vi "OcsWriteFormCsv.vi"() -> ()   [LabVIEW 2018]
panel:
  out "Numeric":i32
  in  "Error in":errorcluster
  out "Error out":errorcluster
  out "W3-TESTER":string
  out "W8-TEXT4":string
  out "W9-OPNAME":string
  out "W0-SN 2":string
  out "SQL Execute":string="SELECT * FROM [FCTDATA].[dbo].[ABF]\nWHERE Barcode = 'P1813J0001'\nORDER BY ID"
  out "W0-SN":string
  out "element":i32
  out "array":string[][](array[string])
  in  ".csv":path
  out "Out":string
  in  "opname":string(combo)="FCT1"
  out "Start Time":dbl
  out "Sec":dbl
  # "Password:Abcd1234* 20220627"
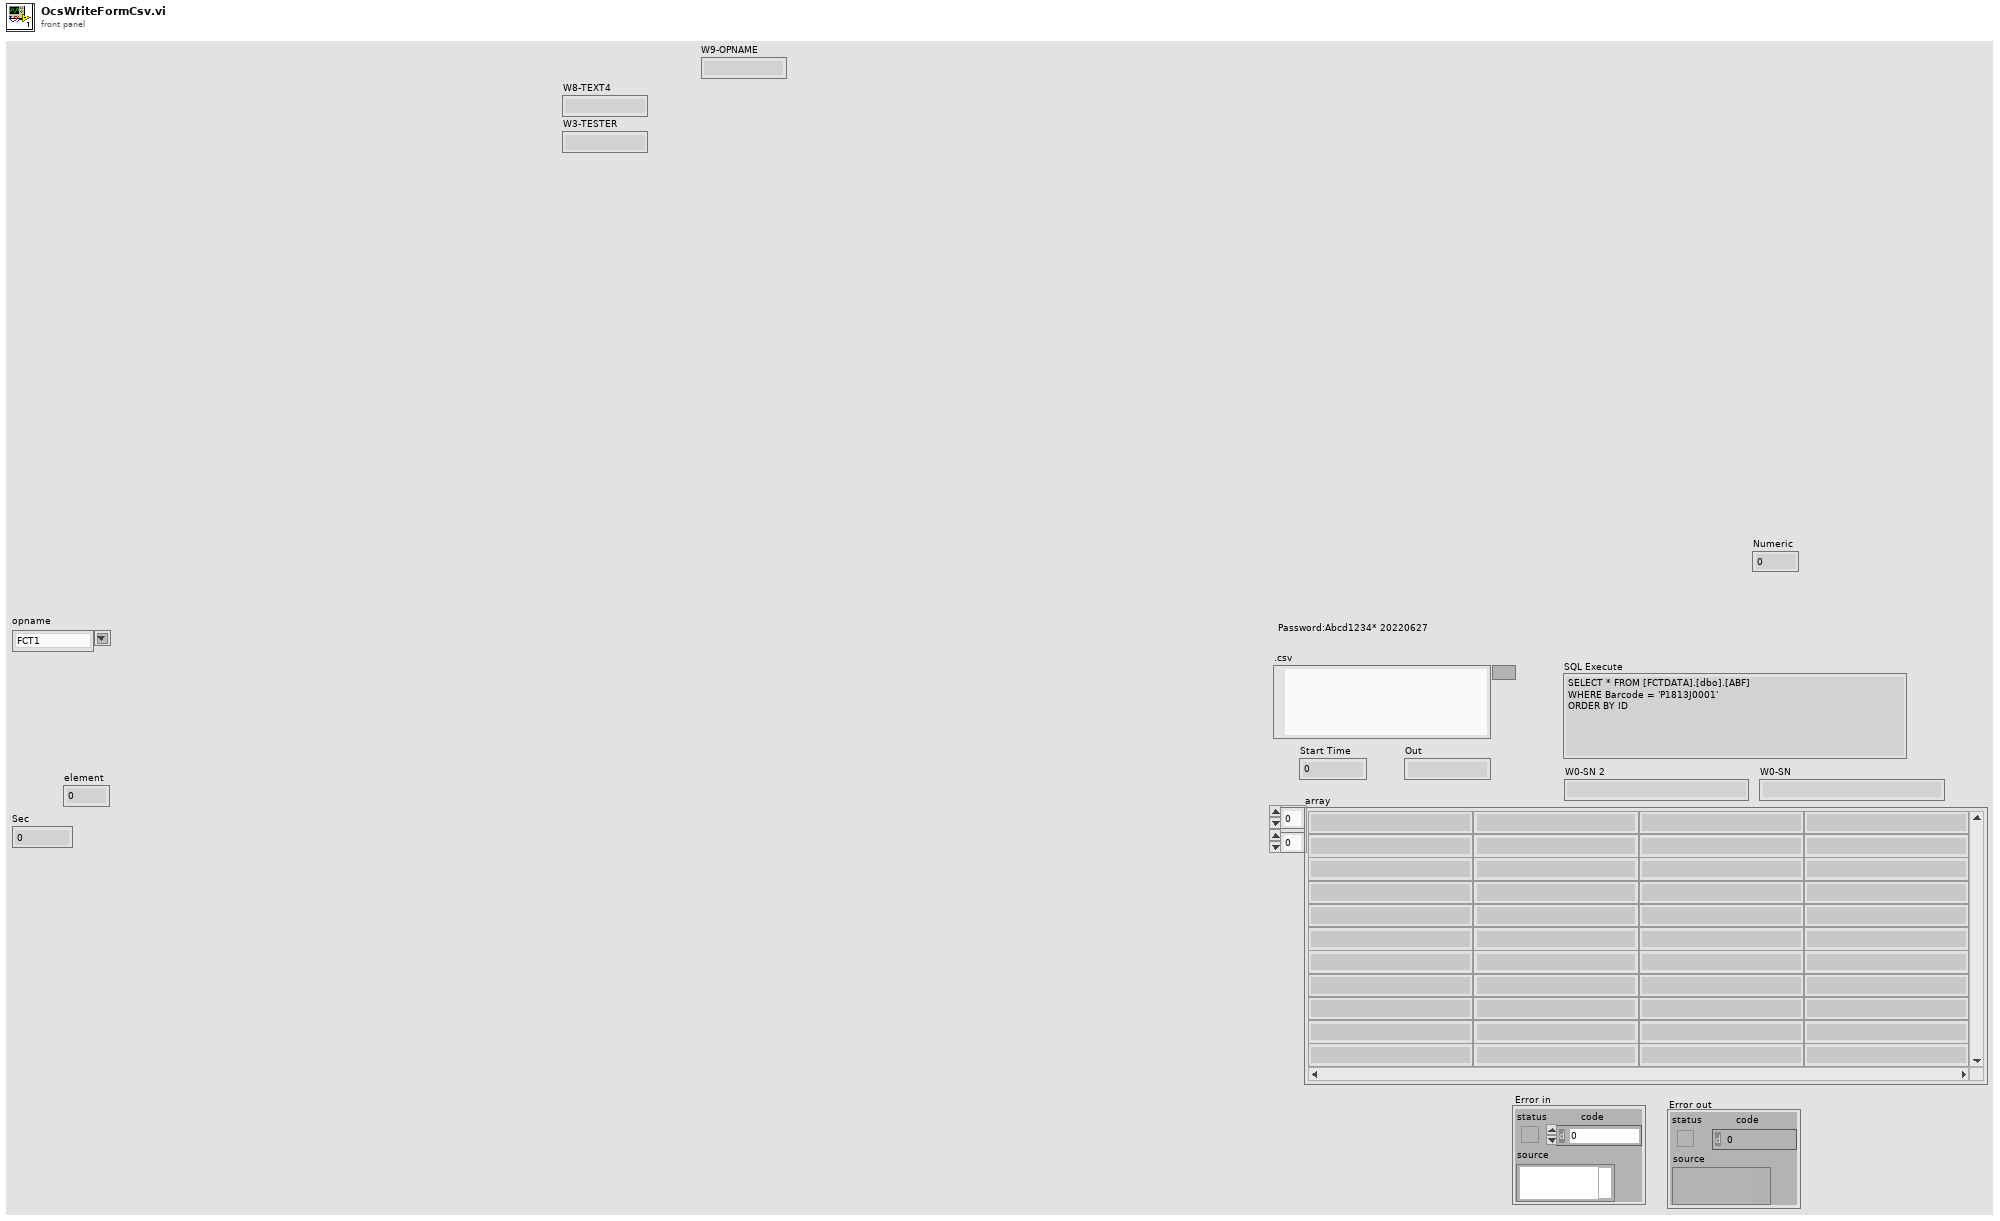
[diagram p1: front panel]
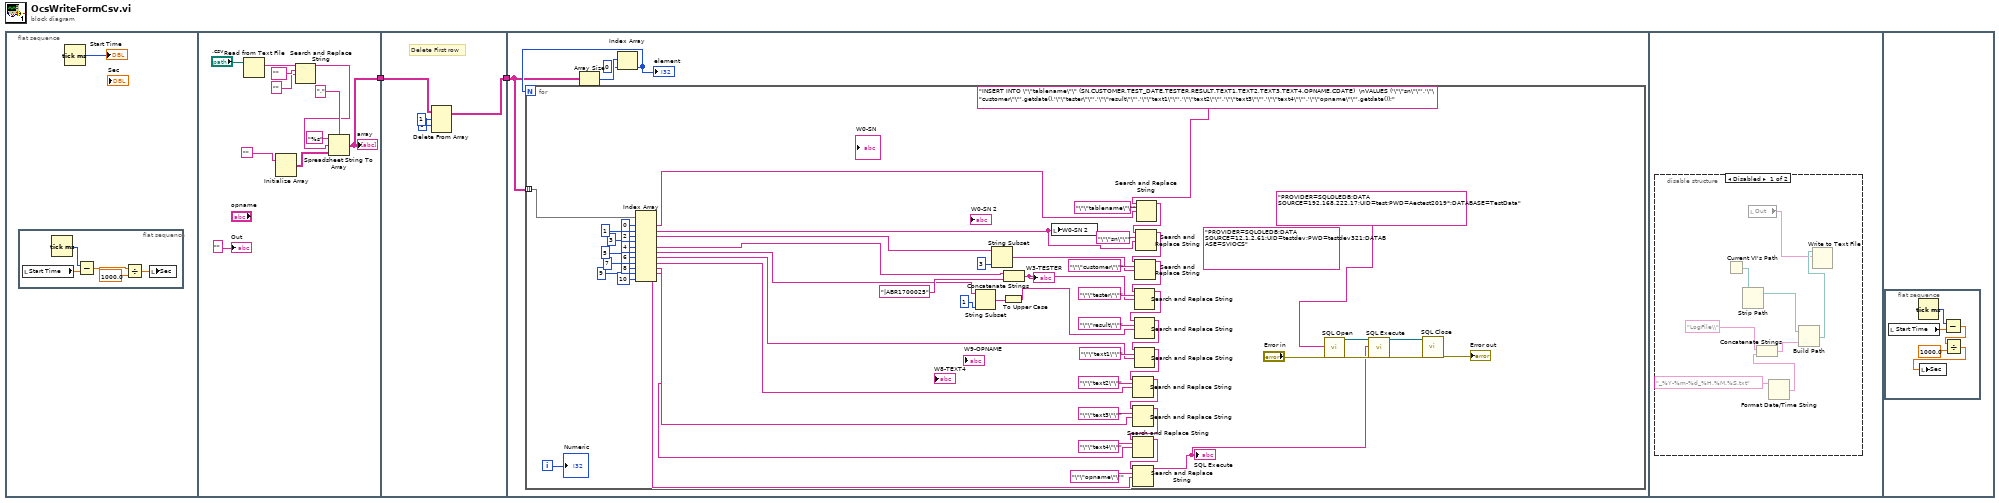
[diagram p0: block diagram]
diagram:
  n1 = flat-sequence {
    tunnel: [w15] -> w2
    tunnel: w2 -> [w23]
    tunnel: [w22] -> w1
    tunnel: w1 -> [w24]
    frame #0 {
      n2 = flat-sequence {
        frame #0 {
          n3 = local read "Start Time"() -> (w7:dbl)
          n4 = Tick Count (ms)() -> (millisecond timer value=w8:u32)
          n5 = Subtract(x=w8, y=w7) -> (x-y=w6:dbl)
          n6 = Divide(x=w6, y=1000.0) -> (x/y=w4:dbl)
          n7 = local write "Sec"(w4) -> ()
        }
      }
      n8 = Tick Count (ms)() -> (millisecond timer value=→"Start Time":u32)
    }
    frame #1 {
      n9 = Read from Text File(file (use dialog)=".csv") -> (text=w12:string)  [unwired: 3 in, 3 out]
      n10 = Initialize Array("") -> (w19:string[][])  [unwired: 2 in]
      n11 = Search and Replace String(input string=w12, search string="﻿" ("replace string (\"\")"), replace string="" ("replace string (\"\")")) -> (result string=w11:string)  [unwired: 5 in, 3 out]
      n12 = Spreadsheet String To Array(delimiter (Tab)="," ("format string"), format string="%s", spreadsheet string=w11, array type (2D Dbl)=w19) -> (array=w15:string[][])
      "array" <- w15
      "Out" <- ""
    }
    frame #2 {
      # "Delete First row"
      n13 = Delete From Array(array=w23, length=1, index (row)=0) -> (array with subset deleted=w22:string[][])  [unwired: 1 in, 1 out]
    }
    frame #3 {
      n14 = Array Size(array=w24) -> (size(s)=w27:i32[])
      n15 = Index Array(array=w27, index=0) -> (element=w25:i32)
      "element" <- w25
      n16 = for {
        N: w25 -> [_]
        tunnel: w24 -> [w85] mode=indexing
        i -> [w29]
        (unwired) "PROVIDER=SQLOLEDB;DATA SOURCE=12.1.2.61;UID=testdev;PWD=testdev321;DATABASE=SVIOCS" ("x")
        n17 = Index Array(array=w85, index #1=0 ("index"), index #2=1 ("index"), index #3=2 ("index"), index #4=3 ("index"), index #5=4 ("index"), index #6=5 ("index"), index #7=6 ("index"), index #8=7 ("index"), index #9=8 ("index"), index #10=9 ("index"), index #11=10 ("index")) -> (element #1=w48:string, element #2=w47:string, element #3=w40:string, element #5=w39:string, element #6=w38:string, element #7=w37:string, element #8=w36:string, element #9=w35:string, element #10=w34:string, element #11=w32:string)  [unwired: 1 out]
        n18 = String Subset(string=w38, length (rest)=1 ("length (rest)")) -> (substring=w73:string)  [unwired: 1 in]
        n19 = String Subset(string=w40, length (rest)=3 ("length (rest)")) -> (substring=w66:string)  [unwired: 1 in]
        n20 = To Upper Case(1:w73) -> (0:w61:string)
        n21 = Concatenate Strings(w39, "|ABR1700025" ("string")) -> (w50:string)
        "W3-TESTER" <- w50
        n22 = local write "W0-SN 2"(w47) -> ()
        n23 = Search and Replace String(input string="INSERT INTO \"\"tablename\"\" (SN,CUSTOMER,TEST_DATE,TESTER,RESULT,TEXT1,TEXT2,TEXT3,TEXT4,OPNAME,CDATE)  \nVALUES ('\"\"sn\"\"','\"\"customer\"\"',getdate(),'\"\"tester\"\"','\"\"result\"\"','\"\"text1\"\"','\"\"text2\"\"','\"\"text3\"\"','\"\"text4\"\"','\"\"opname\"\"',getdate());" ("replace string (\"\")"), search string="\"\"tablename\"\"", replace string=w48) -> (result string=w70:string)  [unwired: 5 in, 3 out]
        n24 = Search and Replace String(input string=w70, search string="\"\"sn\"\"", replace string=w47) -> (result string=w68:string)  [unwired: 5 in, 3 out]
        n25 = Search and Replace String(input string=w68, search string="\"\"customer\"\"", replace string=w66) -> (result string=w65:string)  [unwired: 5 in, 3 out]
        n26 = Search and Replace String(input string=w65, search string="\"\"tester\"\"", replace string=w50) -> (result string=w63:string)  [unwired: 5 in, 3 out]
        n27 = Search and Replace String(input string=w63, search string="\"\"result\"\"", replace string=w61) -> (result string=w60:string)  [unwired: 5 in, 3 out]
        n28 = Search and Replace String(input string=w60, search string="\"\"text1\"\"", replace string=w37) -> (result string=w57:string)  [unwired: 5 in, 3 out]
        n29 = Search and Replace String(input string=w57, search string="\"\"text2\"\"", replace string=w36) -> (result string=w51:string)  [unwired: 5 in, 3 out]
        n30 = Search and Replace String(input string=w51, search string="\"\"text3\"\"", replace string=w35) -> (result string=w52:string)  [unwired: 5 in, 3 out]
        n31 = Search and Replace String(input string=w52, search string="\"\"text4\"\"", replace string=w34) -> (result string=w53:string)  [unwired: 5 in, 3 out]
        n32 = Search and Replace String(input string=w53, search string="\"\"opname\"\"", replace string=w32) -> (result string=w43:string)  [unwired: 5 in, 3 out]
        "SQL Execute" <- w43
        n33 = call "SQL Open.vi"("ConnectionString In"="PROVIDER=SQLOLEDB;DATA SOURCE=192.168.222.17;UID=test;PWD=Aectest2019*;DATABASE=TestData" ("regular expression"), "Error in (no error)"="Error in") -> ("Connection Out"=w45:refnum<k7>, "Error out"=w44:errorcluster)  [unwired: 16 in]
        n34 = call "SQL Execute.vi"("Connection In"=w45, "SQL Query"=w43, "Error in (no error)"=w44) -> ("Connection Out"=w42:refnum<k7>, "Error out"=w41:errorcluster)  [unwired: 15 in]
        n35 = call "SQL Close.vi"("Connection In"=w42, "Error in (no error)"=w41) -> ("Error out"=→"Error out":errorcluster)  [unwired: 17 in]
        "Numeric" <- w29
      }
    }
    frame #4 {
      n36 = disable-structure shown="Disabled" {
        frame Disabled {
          n37 = Current VI's Path() -> (path=w93:path)
          n38 = Strip Path(path=w93) -> (stripped path=w92:path)  [unwired: 1 out]
          n39 = local read "Out"() -> (w87:string)
          n40 = Format Date/Time String(time format string (%c)="_%Y-%m-%d_%H.%M.%S.txt") -> (date/time string=w89:string)  [unwired: 2 in]
          n41 = Concatenate Strings("LogFile\\" ("name or relative path"), w89) -> (w90:string)
          n42 = Build Path(base path=w92, name or relative path=w90) -> (appended path=w88:path)
          n43 = Write to Text File(file (use dialog)=w88, text=w87) -> ()  [unwired: 2 in, 3 out]
        }
        frame Enabled {
        }
      }
    }
    frame #5 {
      n44 = flat-sequence {
        frame #0 {
          n45 = local read "Start Time"() -> (w97:dbl)
          n46 = Tick Count (ms)() -> (millisecond timer value=w98:u32)
          n47 = Subtract(x=w98, y=w97) -> (x-y=w96:dbl)
          n48 = Divide(x=w96, y=1000.0) -> (x/y=w94:dbl)
          n49 = local write "Sec"(w94) -> ()
        }
      }
    }
  }
